vi "Test Waveguide Model.vi"() -> ()   [LabVIEW 2016, in "LockinDAQ.lvclass"]
uses:
  LockinDAQ.lvclass
  <vilib>/Analysis/NI_AALBase.lvlib
panel:
  out "Waveform Graph":dbl[](graph)
  in  "Vsg step (V)":dbl=0.001 format="%#_6p"
  in  "Vsg end (V)":dbl=0.1 format="%#_6p"
  in  "Vsg start (V)":dbl format="%#_6p"
  out "I vs Vsg":cluster{dbl[], dbl[]}(graph)
  in  "V_source (V)":dbl=0.001 format="%#_6p"
  out "G vs Vsg":cluster{dbl[], dbl[]}(graph)
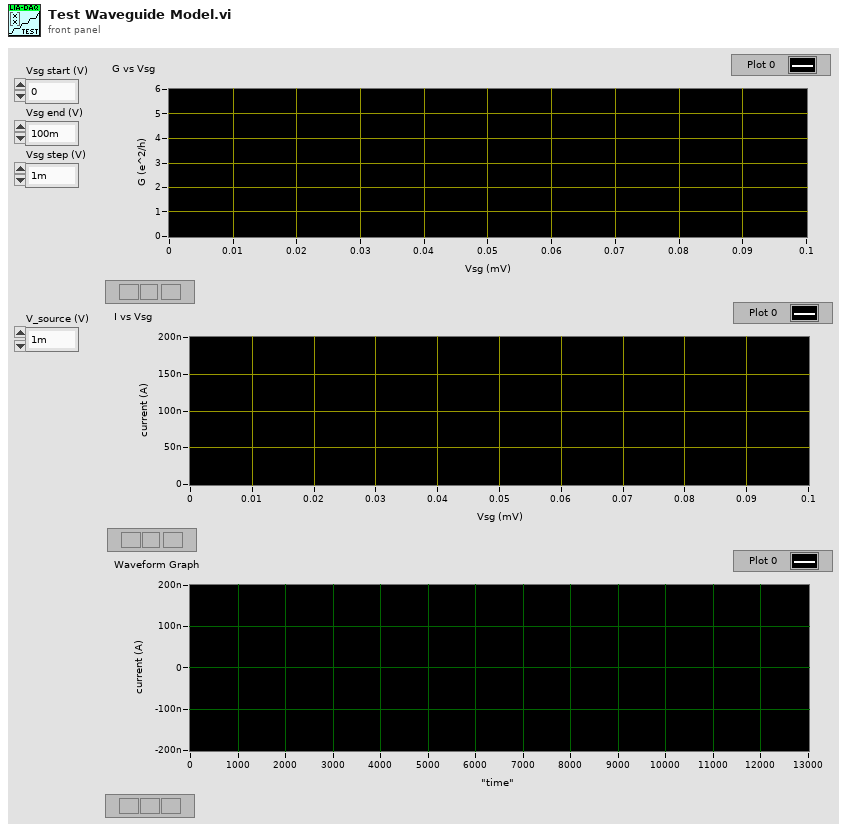
[diagram p1: front panel]
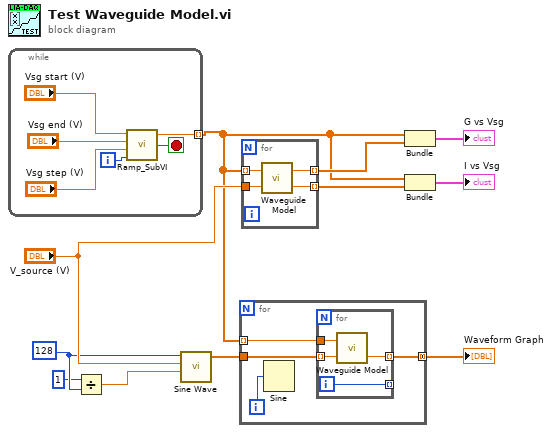
[diagram p0: block diagram]
diagram:
  w4 = 128 ("samples")
  n1 = while {
    tunnel: [w17] -> w2 mode=indexing
    i -> [w13]
    stop <- w12 stop-if-true
    n2 = call <userlib>:"Ramp_SubVI.vi"("index"=w13, "step"="Vsg step (V)", "end"="Vsg end (V)", "start"="Vsg start (V)") -> ("Stop?"=w12:bool, "Numeric"=w17:dbl)  [unwired: 1 in]
  }
  n3 = Divide(x=1, y=w4) -> (x/y=w1:dbl)
  n4 = call <vilib>:"Sine Wave.vi"("samples"=w4, "amplitude"="V_source (V)", "frequency"=w1) -> ("sine wave"=w7:dbl[])  [unwired: 2 in, 2 out]
  n5 = for {
    tunnel: w7 -> [w21]
    tunnel: [w20] -> w6 mode=concatenating
    tunnel: w2 -> [w19] mode=indexing
    i -> [w18]
    n6 = Sine(x=w18) -> ()  [unwired: 1 out]
    n7 = for {
      tunnel: w21 -> [w25] mode=indexing
      tunnel: [w24] -> w20 mode=indexing
      tunnel: [w23] -> _ mode=indexing
      tunnel: w19 -> [w22]
      i -> [w23]
      n8 = call "Waveguide Model.vi"("Vs (V)"=w25, "Vsg (V)"=w22) -> ("I[Vsg] (A)"=w24:dbl)  [unwired: 1 out]
    }
  }
  "Waveform Graph" <- w6
  n9 = for {
    tunnel: w2 -> [w29] mode=indexing
    tunnel: [w27] -> w8 mode=indexing
    tunnel: "V_source (V)" -> [w28]
    tunnel: [w26] -> w9 mode=indexing
    n10 = call "Waveguide Model.vi"("Vs (V)"=w28, "Vsg (V)"=w29) -> ("I[Vsg] (A)"=w26:dbl, "G[Vsg] (e2/h)"=w27:dbl)
  }
  n11 = Bundle(w2, w8) -> (→"G vs Vsg":cluster{dbl[], dbl[]})  [unwired: 1 in]
  n12 = Bundle(w2, w9) -> (→"I vs Vsg":cluster{dbl[], dbl[]})  [unwired: 1 in]
